vi "VISA_1.vi"(6 "delay[ms]":u32=8, 8 "error in":errorcluster, 9 "Enum(txrx)":enum16{"dxrx"}(ring), 10 "wr_buf":string="<03AA1301>", 11 "COM in":string="COM2") -> (0 "error out":errorcluster, 1 "return count":u32, 2 "rx_buf":string="{0FFF}", 3 "COM out":string="COM4")   [LabVIEW 2016]
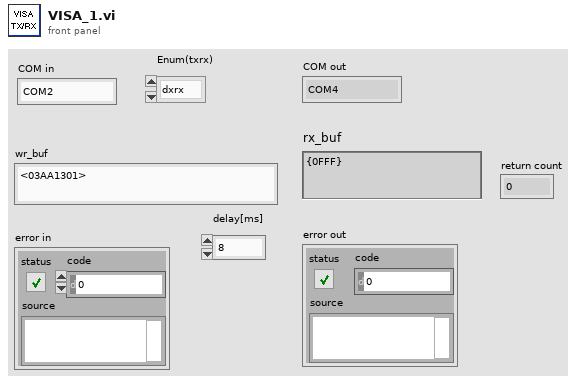
[diagram p1: front panel]
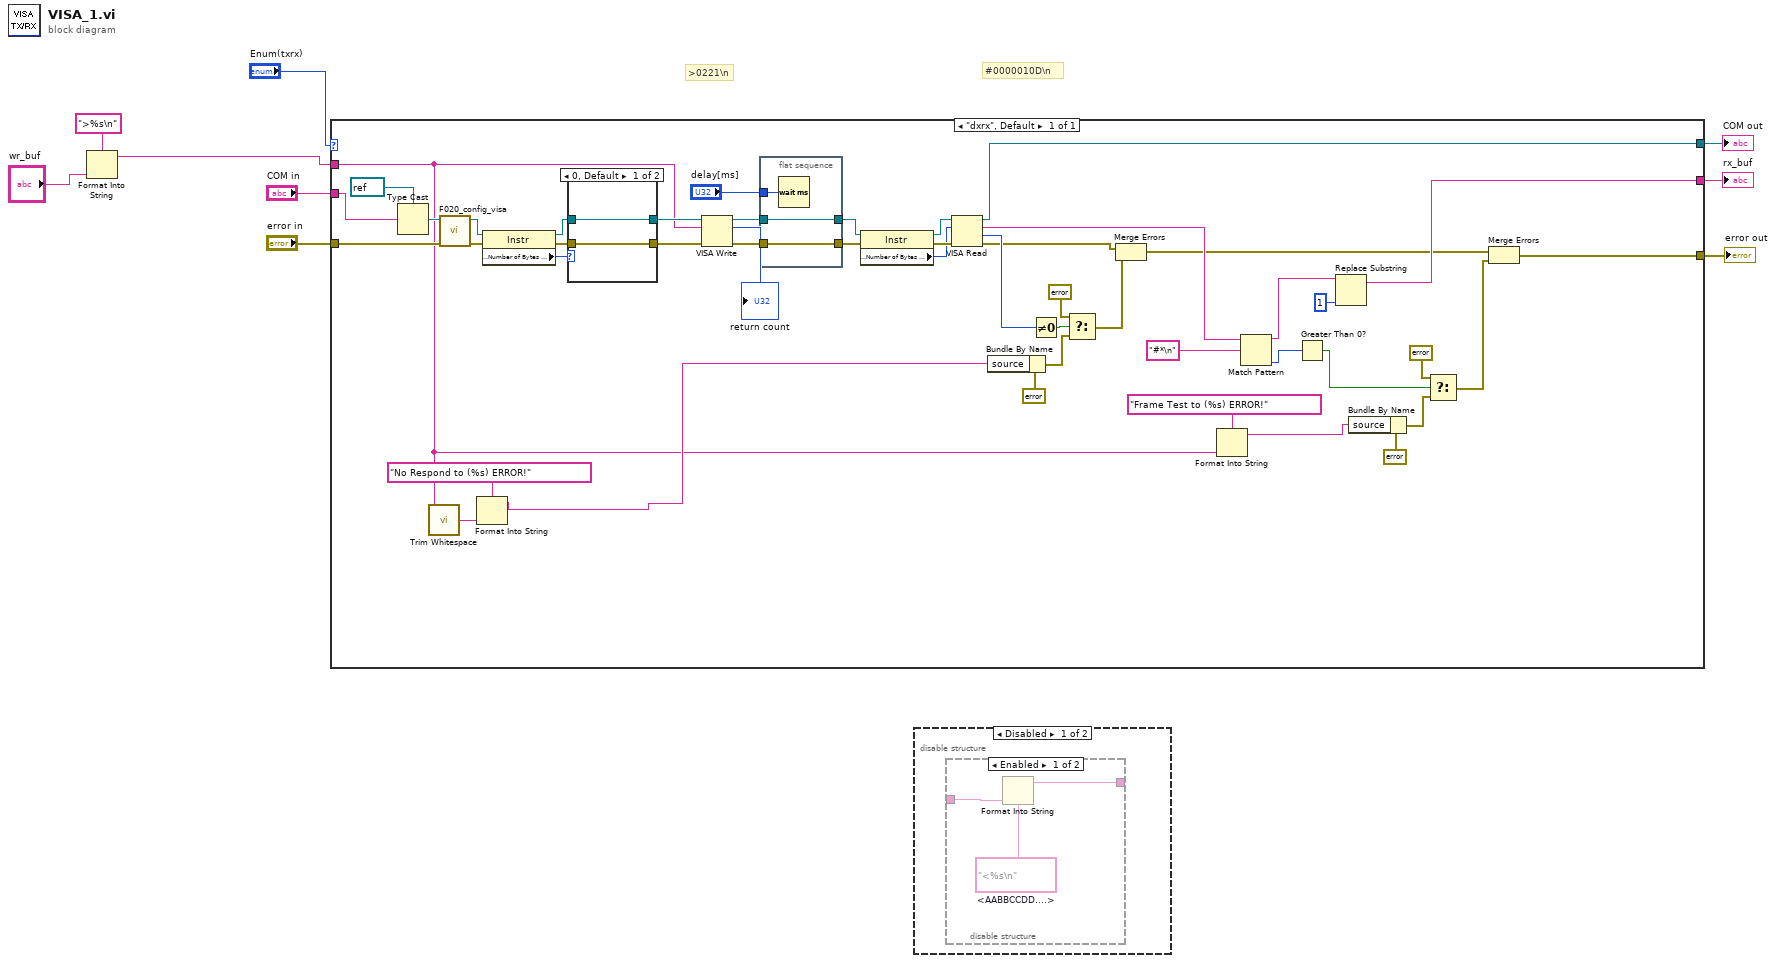
[diagram p0: block diagram]
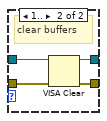
[diagram p4: hidden frame]
diagram:
  # "#0000010D\\n"
  # ">0221\\n"
  n1 = Format Into String(format string=">%s\n" ("source"), "wr_buf") -> (resulting string=w1:string)  [unwired: 2 in, 1 out]
  n2 = case shown="\"dxrx\", Default" "Enum(txrx)" {
    tunnel: [w56] -> w9
    tunnel: "error in" -> [w37]
    tunnel: "COM in" -> [w45]
    tunnel: w1 -> [w19]
    tunnel: [w29] -> w6
    tunnel: [w12] -> w4
    frame "dxrx", Default {
      n3 = Type Cast(type=refnum<visa-resource-name> refnum ("VISA resource name out"), x=w45) -> (*(type *) &x=w40:refnum<visa-resource-name>)
      n4 = call <vilib>:"Trim Whitespace.vi"("string"=w19) -> ("trimmed string"=w11:string)  [unwired: 1 in]
      n5 = call "F020_config_visa.vi"("error in (no error)"=w37, "VISA Refnum in"=w40) -> ("error out"=w38:errorcluster, "VISA Refnum out"=w39:refnum<visa-resource-name>)  [unwired: 8 in]
      n6 = Format Into String(format string="No Respond to (%s) ERROR!" ("source"), w11) -> (resulting string=w22:string)  [unwired: 2 in, 1 out]
      n7 = property class="Instr"(reference=w39, error in=w38) -> (reference out=w43:refnum<visa-resource-name>, error out=w41:errorcluster, "Serial Settings:Number of Bytes at Serial Port"=w42:u32)
      n8 = case shown="0, Default" w42 {
        tunnel: [w57 w62] -> w47
        tunnel: w41 -> [w58 w61]
        tunnel: [w58 w60] -> w46
        tunnel: w43 -> [w57 w59]
        frame 0, Default {
        }
        frame 1.. {
          # "clear buffers"
          n9 = VISA Clear(VISA resource name=w59, error in (no error)=w61) -> (VISA resource name out=w62:refnum<visa-resource-name>, error out=w60:errorcluster)
        }
      }
      n10 = VISA Write(VISA resource name=w47, write buffer=w19, error in (no error)=w46) -> (VISA resource name out=w53:refnum<visa-resource-name>, return count=→"return count":u32, error out=w55:errorcluster)
      n11 = flat-sequence {
        tunnel: w55 -> [w64]
        tunnel: [w64] -> w54
        tunnel: w53 -> [w63]
        tunnel: [w63] -> w52
        tunnel: "delay[ms]" -> [w65]
        frame #0 {
          n12 = Wait (ms)(milliseconds to wait=w65) -> ()  [unwired: 1 out]
        }
      }
      n13 = property class="Instr"(reference=w52, error in=w54) -> (reference out=w50:refnum<visa-resource-name>, error out=w49:errorcluster, "Serial Settings:Number of Bytes at Serial Port"=w48:u32)
      n14 = VISA Read(VISA resource name=w50, byte count=w48, error in (no error)=w49) -> (VISA resource name out=w56:refnum<visa-resource-name>, read buffer=w30:string, return count=w34:u32, error out=w27:errorcluster)
      n15 = Bundle By Name(cluster=errorcluster {"status"=TRUE, "code"=-8000, "source"="No Respond to (%s) ERROR!"} ("f"), "source"=w22) -> (w21:errorcluster)
      n16 = Not Equal To 0?(x=w34) -> (x != 0?=w33:bool)
      n17 = Select(t=errorcluster {"status"=FALSE, "code"=0, "source"=""}, s=w33, f=w21) -> (s? t:f=w26:errorcluster)
      n18 = Merge Errors(w27, w26) -> (w24:errorcluster)
      n19 = Format Into String(format string="Frame Test to (%s) ERROR!" ("source"), w19) -> (resulting string=w14:string)  [unwired: 2 in, 1 out]
      n20 = Match Pattern(string=w30, regular expression="#*\n") -> (before substring=w31:string, offset past match=w35:i32)  [unwired: 1 in, 2 out]
      n21 = Greater Than 0?(x=w35) -> (x > 0?=w15:bool)
      n22 = Replace Substring(2:1 ("length (len. of substring)"), 5:w31) -> (1:w29:string)  [unwired: 2 in, 1 out]
      n23 = Bundle By Name(cluster=errorcluster {"status"=TRUE, "code"=-8000, "source"="No Respond to (%s) ERROR!"} ("f"), "source"=w14) -> (w18:errorcluster)
      n24 = Select(t=errorcluster {"status"=FALSE, "code"=0, "source"=""}, s=w15, f=w18) -> (s? t:f=w13:errorcluster)
      n25 = Merge Errors(w24, w13) -> (w12:errorcluster)
    }
  }
  "rx_buf" <- w6
  "COM out" <- w9
  "error out" <- w4
  n26 = disable-structure shown="Disabled" {
    frame Disabled {
      n27 = disable-structure shown="Enabled" {
        disable-tunnel: _ -> [w68 w69]
        disable-tunnel: [w66 w69] -> _
        frame Enabled {
          w67 = "<%s\n"  # <AABBCCDD....>
          n28 = Format Into String(format string=w67, w68) -> (resulting string=w66:string)  [unwired: 2 in, 1 out]
        }
        frame Disabled {
        }
      }
    }
    frame Enabled {
    }
  }
